vi "SUB_READ_COM1_FindString_timeout.vi"(4 "Find this String":string, 5 "Timeout Seccond":dbl, 6 "Begin time":dbl, 7 "duplicate VISA resource name 2":refnum<visa-resource-name>) -> (1 "Output String":string, 2 "spent seconds":dbl, 3 "Found String":bool)   [LabVIEW 2011]
panel:
  out "String":string
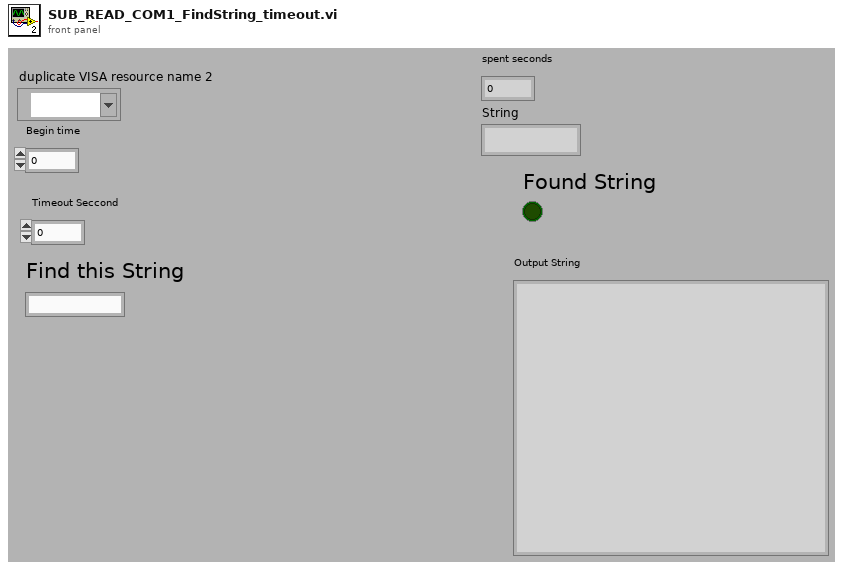
[diagram p1: front panel]
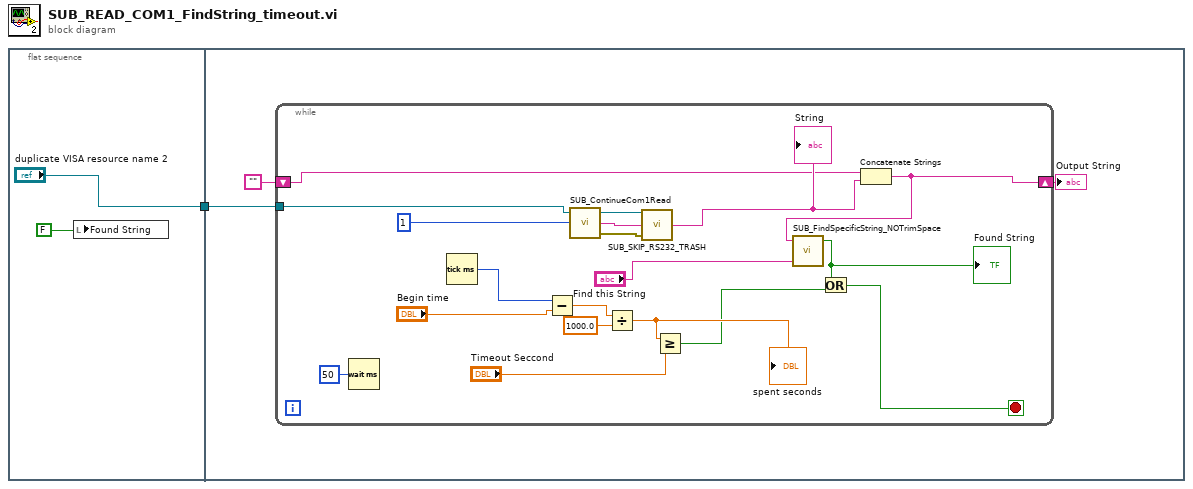
[diagram p0: block diagram]
diagram:
  n1 = flat-sequence {
    tunnel: ["duplicate VISA resource name 2"] -> w1
    tunnel: w1 -> [w4]
    frame #0 {
      n2 = local write "Found String"(FALSE) -> ()
    }
    frame #1 {
      n3 = while {
        shift-right: [w9] -> w5
        shift-left: "" -> [w12]
        tunnel: w4 -> [w8]
        stop <- w15 stop-if-true
        n4 = Wait (ms)(milliseconds to wait=u32 50) -> ()  [unwired: 1 out]
        n5 = Tick Count (ms)() -> (millisecond timer value=w11:u32)
        n6 = Subtract(x=w11, y="Begin time") -> (x-y=w21:dbl)
        n7 = call "SUB_ContinueCom1Read.vi"("Numeric"=1, "duplicate VISA resource name 2"=w8) -> ("error out"=w23:errorcluster, "String"=w24:string, "duplicate VISA resource name"=w25:refnum<visa-resource-name>)  [unwired: 1 in]
        n8 = Divide(x=w21, y=1000.0) -> (x/y=w19:dbl)
        "spent seconds" <- w19
        n9 = call "SUB_SKIP_RS232_TRASH.vi"("error out 2"=w23, "read buffer"=w24, "duplicate VISA resource name 2"=w25) -> ("String"=w13:string)  [unwired: 2 out]
        "String" <- w13
        n10 = Greater Or Equal?(x=w19, y="Timeout Seccond") -> (x >= y?=w16:bool)
        n11 = Concatenate Strings(w12, w13) -> (w9:string)
        n12 = call "SUB_FindSpecificString_NOTrimSpace.vi"("Find this String"="Find this String", "String data"=w9) -> ("Found"=w17:bool)  [unwired: 2 in, 1 out]
        "Found String" <- w17
        n13 = Or(x=w17, y=w16) -> (x .or. y?=w15:bool)
      }
      "Output String" <- w5
    }
  }
